vi "Set Events Q.vi"(10 "Events Q":refnum<class "MessageQ.lvclass">, 11 "VolatusAPI in":refnum<class "VolatusAPI.lvclass">) -> (3 "VolatusAPI out":refnum<class "VolatusAPI.lvclass">)   [LabVIEW 2020, in "Volatus.lvlib" / "VolatusAPI.lvclass"]
uses:
  VolatusAPI.lvclass
  MessageQ/MessageQ.lvclass
  VolatusAPI.lvclass/VolatusAPI.ctl
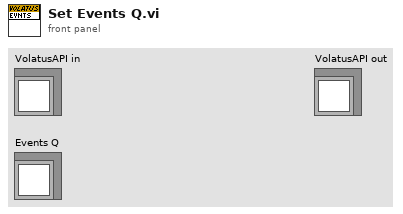
[diagram p1: front panel]
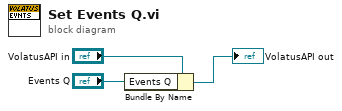
[diagram p0: block diagram]
diagram:
  n1 = Bundle By Name(cluster="VolatusAPI in", "Events Q"="Events Q") -> (→"VolatusAPI out":refnum<class "VolatusAPI.lvclass">)
